vi "ManualLauncher.vi"   [LabVIEW 2012]
uses:
  State_Machine_Enum.ctl
  Robot Global Data.vi
types:
  T1 = typedef "State_Machine_Enum.ctl" = enum16{"Init", "Idle", "Start", "Do", "Stop"}
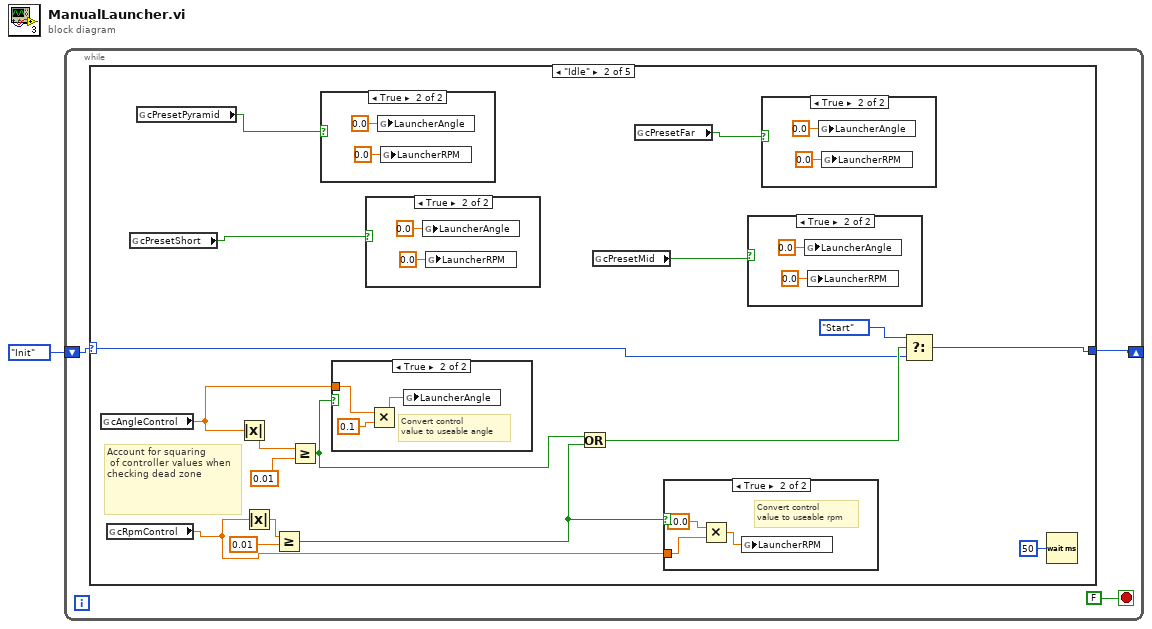
[diagram p0: block diagram]
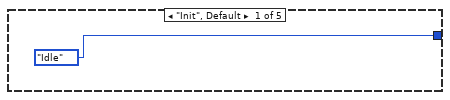
[diagram p2: hidden frame]
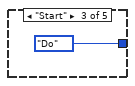
[diagram p9: hidden frame]
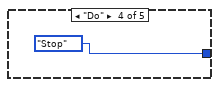
[diagram p10: hidden frame]
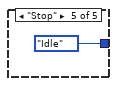
[diagram p11: hidden frame]
diagram:
  n1 = while {
    shift-right: [w2] -> _
    shift-left: State_Machine_Enum."Init" ("State") -> [w4]
    stop <- FALSE stop-if-true
    n2 = case shown="\"Idle\"" w4 {
      selector: w4 -> [_ w13 _ _ _]
      tunnel: [State_Machine_Enum."Idle" ("State") w22 State_Machine_Enum."Do" ("State") State_Machine_Enum."Stop" ("State") State_Machine_Enum."Idle" ("State")] -> w2
      frame "Init", Default {
      }
      frame "Idle" {
        # "Account for squaring\n of controller values when checking dead zone"
        n3 = global read "Robot Global Data.vi" "cAngleControl"() -> (w10:dbl)
        n4 = global read "Robot Global Data.vi" "cRpmControl"() -> (w8:dbl)
        n5 = global read "Robot Global Data.vi" "cPresetShort"() -> (w17:bool)
        n6 = global read "Robot Global Data.vi" "cPresetPyramid"() -> (w18:bool)
        n7 = Absolute Value(x=w10) -> (abs(x)=w9:dbl)
        n8 = Absolute Value(x=w8) -> (abs(x)=w7:dbl)
        n9 = Greater Or Equal?(x=w7, y=0.01) -> (x >= y?=w14:bool)
        n10 = Greater Or Equal?(x=w9, y=0.01) -> (x >= y?=w12:bool)
        n11 = case shown="True" w18 {
          frame False {
          }
          frame True {
            n12 = global write "Robot Global Data.vi" "LauncherAngle"(0.0 ("LauncherAngle")) -> ()
            n13 = global write "Robot Global Data.vi" "LauncherRPM"(0.0 ("LauncherRPM")) -> ()
          }
        }
        n14 = case shown="True" w12 {
          tunnel: w10 -> [_ w25]
          frame False {
          }
          frame True {
            # "Convert control\nvalue to useable angle"
            n15 = Multiply(x=w25, y=0.1) -> (x*y=w23:dbl)
            n16 = global write "Robot Global Data.vi" "LauncherAngle"(w23) -> ()
          }
        }
        n17 = case shown="True" w17 {
          frame False {
          }
          frame True {
            n18 = global write "Robot Global Data.vi" "LauncherAngle"(0.0 ("LauncherAngle")) -> ()
            n19 = global write "Robot Global Data.vi" "LauncherRPM"(0.0 ("LauncherRPM")) -> ()
          }
        }
        n20 = Or(x=w12, y=w14) -> (x .or. y?=w19:bool)
        n21 = global read "Robot Global Data.vi" "cPresetMid"() -> (w15:bool)
        n22 = global read "Robot Global Data.vi" "cPresetFar"() -> (w16:bool)
        n23 = case shown="True" w14 {
          tunnel: w8 -> [_ w28]
          frame False {
          }
          frame True {
            # "Convert control\nvalue to useable rpm"
            n24 = Multiply(x=10.0, y=w28) -> (x*y=w27:dbl)
            n25 = global write "Robot Global Data.vi" "LauncherRPM"(w27) -> ()
          }
        }
        n26 = case shown="True" w15 {
          frame False {
          }
          frame True {
            n27 = global write "Robot Global Data.vi" "LauncherAngle"(0.0 ("LauncherAngle")) -> ()
            n28 = global write "Robot Global Data.vi" "LauncherRPM"(0.0 ("LauncherRPM")) -> ()
          }
        }
        n29 = case shown="True" w16 {
          frame False {
          }
          frame True {
            n30 = global write "Robot Global Data.vi" "LauncherAngle"(0.0 ("LauncherAngle")) -> ()
            n31 = global write "Robot Global Data.vi" "LauncherRPM"(0.0 ("LauncherRPM")) -> ()
          }
        }
        n32 = Select(t=State_Machine_Enum."Start" ("State"), s=w19, f=w13) -> (s? t:f=w22:T1)
        n33 = Wait (ms)(milliseconds to wait=u32 50) -> ()  [unwired: 1 out]
      }
      frame "Start" {
      }
      frame "Do" {
      }
      frame "Stop" {
      }
    }
  }
